vi "initialize python session.vi"(8 "error in (no error)":errorcluster, 10 "Optional Path to Python.exe":path=path "", 11 "Save Image in":refnum<class "Save Image.lvclass">) -> (0 "error out":errorcluster, 3 "Save Image out":refnum<class "Save Image.lvclass">)   [LabVIEW 2018, in "Save Image.lvclass"]
uses:
  Save Image.lvclass
  Save Image.lvclass/Save Image.ctl
  Python Toolkit/Python Toolkit.lvclass/Python Toolkit.ctl
  Python Toolkit/Python Toolkit.lvclass
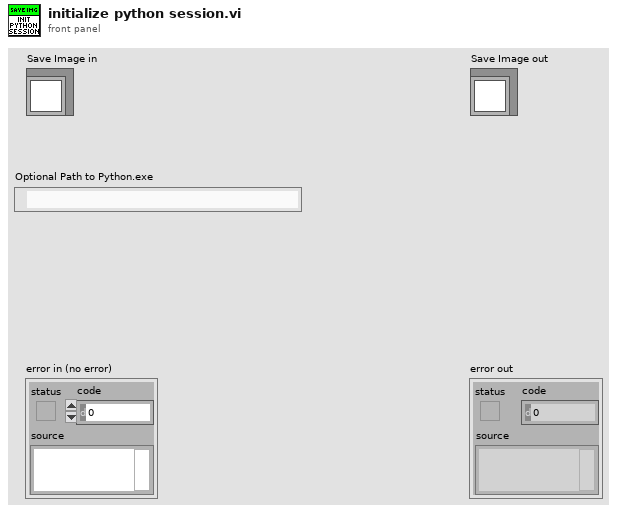
[diagram p1: front panel]
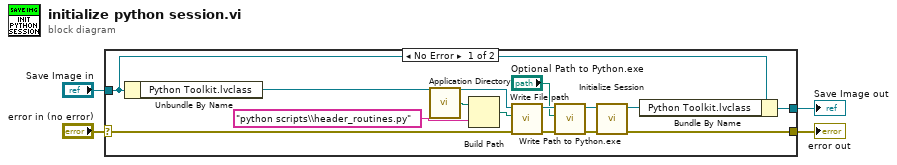
[diagram p0: block diagram]
diagram:
  n1 = case shown="No Error" "error in (no error)" {
    selector: "error in (no error)" -> [w11 w20]
    tunnel: [w10 w20] -> w3
    tunnel: [w15 w19] -> w1
    tunnel: "Save Image in" -> [w14 w19]
    frame No Error {
      n2 = Unbundle By Name(w14) -> ("Python Toolkit.lvclass"=w17:refnum<class "Python Toolkit.lvclass">)
      n3 = call <vilib>:"Application Directory.vi"() -> ("Application Directory"=w12:path)
      n4 = Build Path(base path=w12, name or relative path="python scripts\\header_routines.py") -> (appended path=w16:path)
      n5 = call "Write File path.vi"("error in (no error)"=w11, "File path"=w16, "Python Toolkit in"=w17) -> ("error out"=w9:errorcluster, "Python Toolkit out"=w6:refnum<class "Python Toolkit.lvclass">)  [unwired: 7 in]
      n6 = call-dynamic "Write Path to Python.exe.vi"("error in (no error)"=w9, "Optional Path to Python.exe"="Optional Path to Python.exe", "Python Toolkit in"=w6) -> ("error out"=w8:errorcluster, "Python Toolkit out"=w7:refnum<class "Python Toolkit.lvclass">)  [unwired: 7 in]
      n7 = call "Initialize Session.vi"("error in (no error)"=w8, "Python Toolkit in"=w7) -> ("error out"=w10:errorcluster, "Python Toolkit out"=w18:refnum<class "Python Toolkit.lvclass">)  [unwired: 8 in]
      n8 = Bundle By Name(cluster=w14, "Python Toolkit.lvclass"=w18) -> (w15:refnum<class "Save Image.lvclass">)
    }
    frame Error {
    }
  }
  "error out" <- w3
  "Save Image out" <- w1
